vi "Sandbox.vi"() -> ()   [LabVIEW 2022 SP3]
uses:
  <vilib>/Utility/file.llb/Read Delimited Spreadsheet (string).vi
panel:
  out "filenames":string[](array[string])
  out "return value 2":string[](array[string])
  out "return value":string[][](array[string])
  out "subarray":string[](array[string])
  out "Array":string[](array[string])
  in  "file path (dialog if empty)":path
  in  "Reset":bool
  in  "Stop":bool
  out "Elapsed Time (s)":dbl
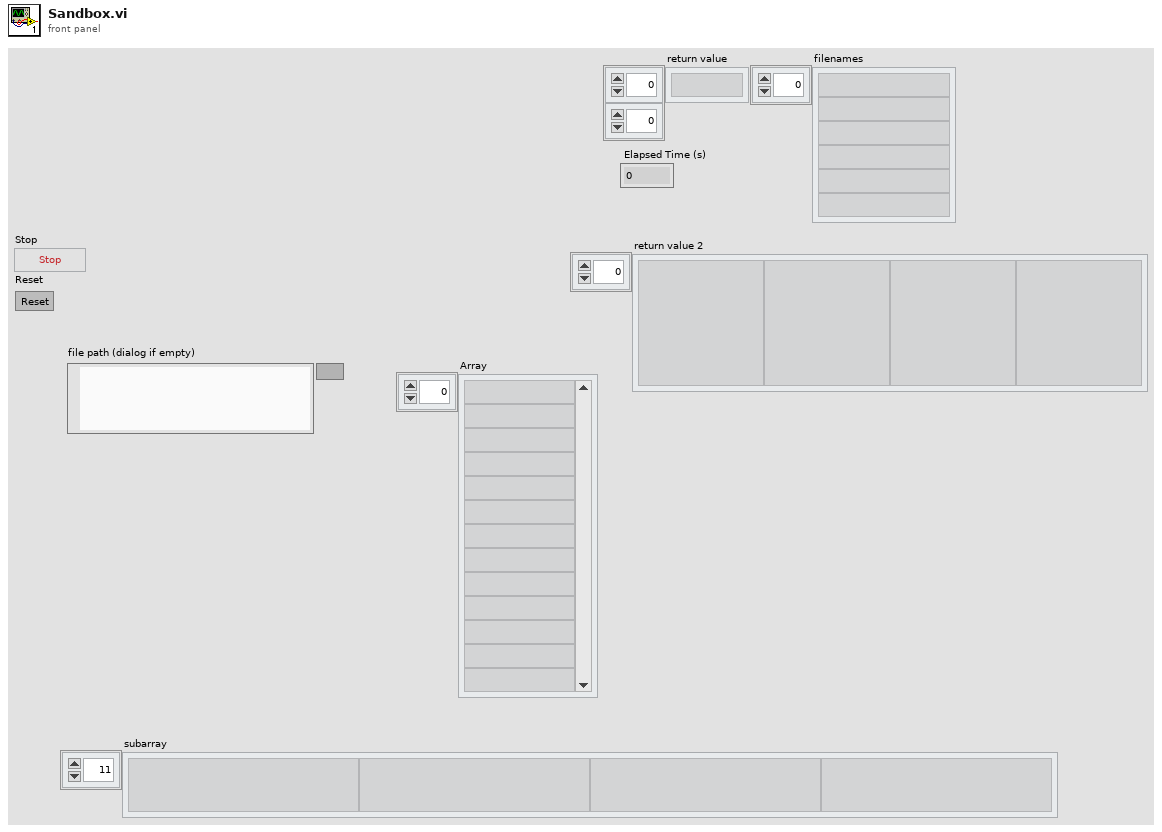
[diagram p1: front panel]
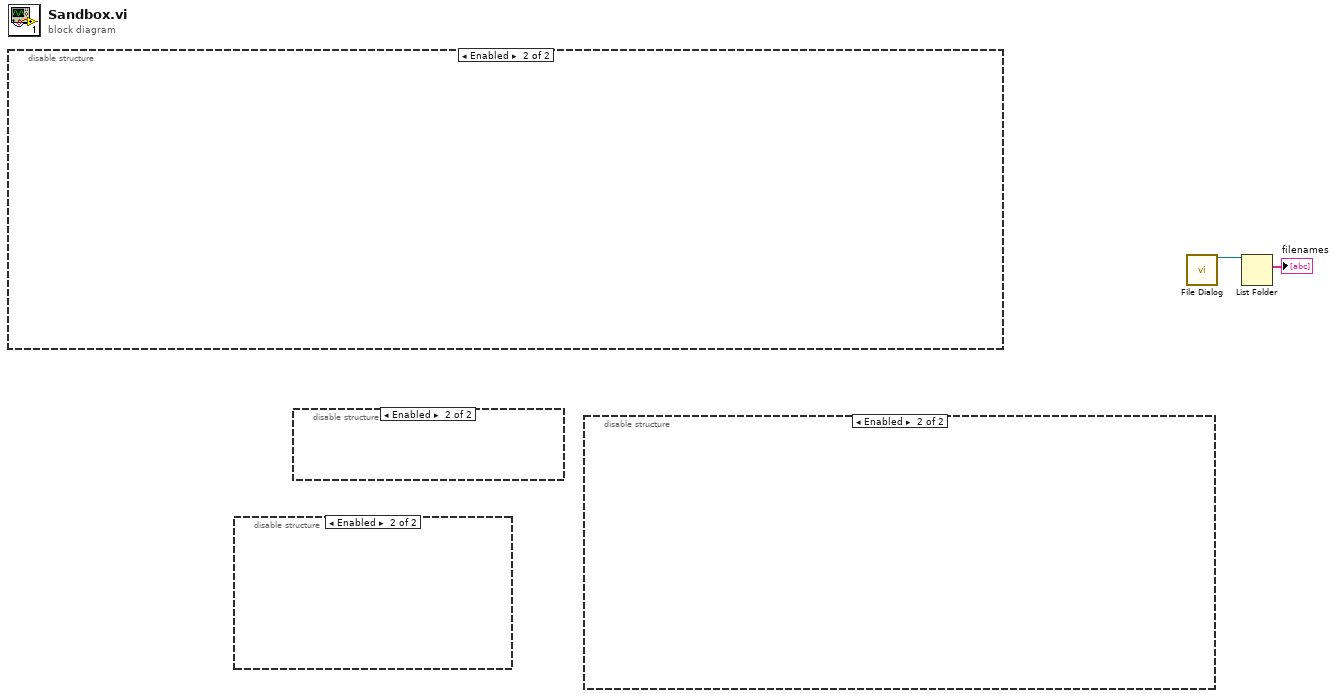
[diagram p0: block diagram]
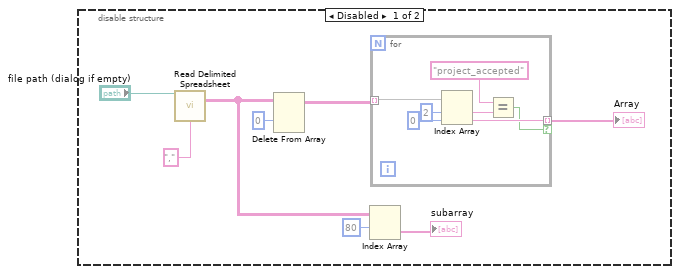
[diagram p2: hidden frame]
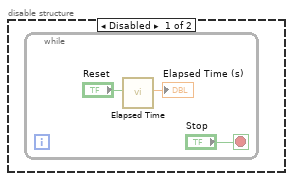
[diagram p3: hidden frame]
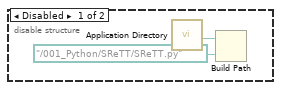
[diagram p4: hidden frame]
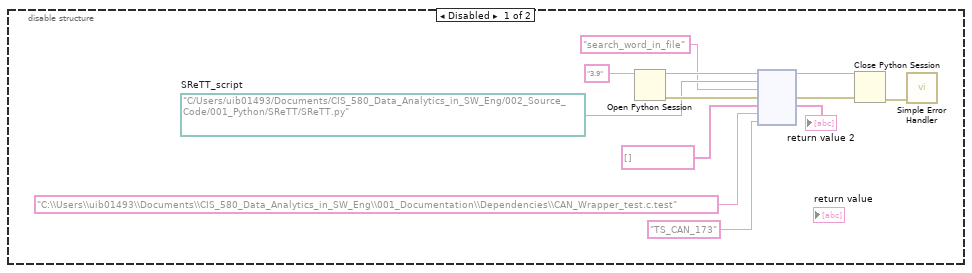
[diagram p5: hidden frame]
diagram:
  n1 = disable-structure shown="Enabled" {
    frame Disabled {
      w8 = path "C:/Users/uib01493/Documents/CIS_580_Data_Analytics_in_SW_Eng/002_Source_Code/001_Python/SReTT/SReTT.py"  # SReTT_script
      n2 = Open Python Session(python version="3.9" ("Python version")) -> (session out=w12:refnum<k35>, error out=w10:errorcluster)  [unwired: 2 in]
      n3 = node(w12, w8, "search_word_in_file" ("function name"), w10, string[] [], "C:\\Users\\uib01493\\Documents\\CIS_580_Data_Analytics_in_SW_Eng\\001_Documentation\\Dependencies\\CAN_Wrapper_test.c.test" ("function name"), "TS_CAN_173" ("function name")) -> (w11:refnum<k35>, w9:errorcluster, →"return value 2":string[])  [unwired: 2 in, 2 out]
      n4 = Close Python Session(session in=w11, error in=w9) -> (11:w13:errorcluster)
      n5 = call <vilib>:"Simple Error Handler.vi"("error in (no error)"=w13) -> ()  [unwired: 4 in, 5 out]
    }
    frame Enabled {
    }
  }
  n6 = disable-structure shown="Enabled" {
    frame Disabled {
      n7 = while {
        stop <- "Stop" stop-if-true
        n8 = call "Elapsed Time"("Reset"="Reset") -> ("Elapsed Time (s)"=→"Elapsed Time (s)":dbl)  [unwired: 11 in, 7 out]
      }
    }
    frame Enabled {
    }
  }
  n9 = disable-structure shown="Enabled" {
    frame Disabled {
      n10 = call <vilib>:"Application Directory.vi"() -> ("Application Directory"=w19:path)
      n11 = Build Path(base path=w19, name or relative path=path "../001_Python/SReTT/SReTT.py") -> ()  [unwired: 1 out]
    }
    frame Enabled {
    }
  }
  n12 = disable-structure shown="Enabled" {
    frame Disabled {
      n13 = call-poly <vilib>:"Read Delimited Spreadsheet.vi"("file path (dialog if empty)"="file path (dialog if empty)", "delimiter (\\t)"="," ("delimiter (\\t)")) -> ("all rows"=w22:string[][])  [unwired: 8 in, 5 out]
      n14 = Delete From Array(array=w22, index (row)=0) -> (array with subset deleted=w24:string[][])  [unwired: 2 in, 1 out]
      n15 = Index Array(array=w22, index (row)=80) -> (element=→"subarray":string[])  [unwired: 1 in]
      n16 = for {
        tunnel: w24 -> [w34] mode=indexing
        tunnel: [w29] -> w23 mode=indexing if=w28
        n17 = Index Array(array=w34, index #1=2 ("index"), index #2=0 ("index")) -> (element #1=w31:string, element #2=w29:string)
        n18 = Equal?(x="project_accepted" ("y"), y=w31) -> (x = y?=w28:bool)
      }
      "Array" <- w23
    }
    frame Enabled {
    }
  }
  n19 = call "File Dialog"() -> ("selected path"=w2:path)  [unwired: 12 in, 3 out]
  n20 = List Folder(path=w2) -> (filenames=→"filenames":string[])  [unwired: 3 in, 3 out]
